vi "checkFinishBallChallengePlayVSS.vi"(8 "error in (no error)":errorcluster, 9 "last command_interpreted":T1, 10 "Game in":refnum<class "Game.lvclass">, 11 "BallChallengePlayVSS in":refnum<class "BallChallengePlayVSS.lvclass">) -> (0 "error out":errorcluster, 2 "Boolean":bool, 3 "BallChallengePlayVSS out":refnum<class "BallChallengePlayVSS.lvclass">)   [LabVIEW 2018, in "BallChallengePlayVSS.lvclass"]
uses:
  BallChallengePlayVSS.lvclass
  Game_class/Game.lvclass
  Referee_class/command_interpreted.ctl
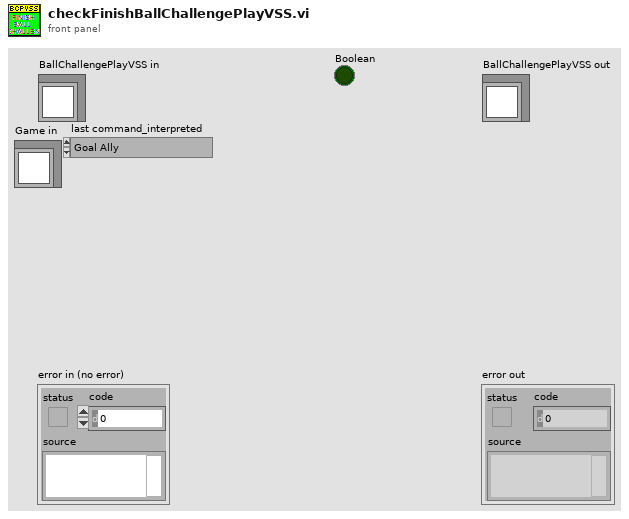
[diagram p1: front panel]
types:
  T1 = typedef "command_interpreted.ctl" = enum16{"Goal Ally", "Goal Enemy", "Ball Placement Enemy", "Ball Placement Ally", "Normal Half Time", "Extra Time  Break", "Extra Half Time", "None", "Post Game", "PKA Normal Start", "Prepare Kickoff Ally", "PKE Normal Start", "Prepare Kickoff Enemy", "Force Start", "Halt", "Timeout", "Prepare Penalty Ally", "Prepare Penalty Enemy", "PPA NormalStart", "PPE Normal Start", "Indirect Free Ally", "Direct Free Enemy", "Direct Free Ally", "Indirect Free Enemy", "Stop"}
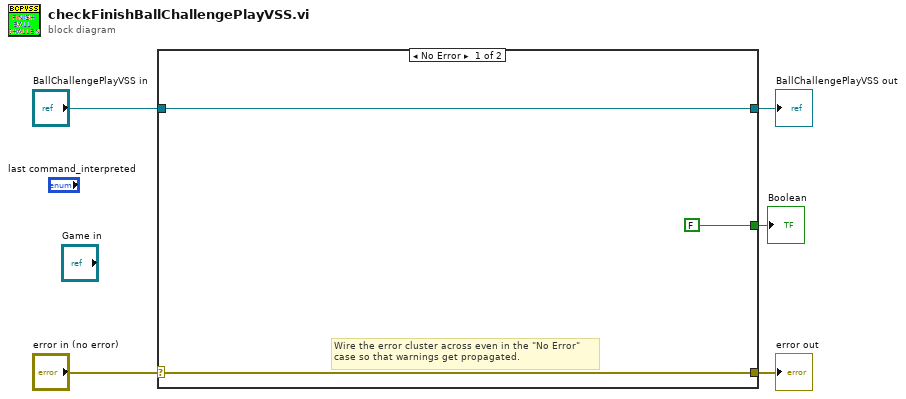
[diagram p0: block diagram]
diagram:
  n1 = case shown="No Error" "error in (no error)" {
    selector: "error in (no error)" -> [w7 w10]
    tunnel: [w7 w10] -> w4
    tunnel: [w8 w9] -> w2
    tunnel: "BallChallengePlayVSS in" -> [w8 w9]
    tunnel: [FALSE _] -> w1
    frame No Error {
      # "Wire the error cluster across even in the \"No Error\"\ncase so that warnings get propagated."
    }
    frame Error {
    }
  }
  "error out" <- w4
  "BallChallengePlayVSS out" <- w2
  "Boolean" <- w1
